vi "Delete TEMP FP Labels.vi"(8 "error in":errorcluster, 11 "owner VI":refnum<vi>) -> (0 "error out":errorcluster, 1 "labels found":i32, 3 "owner VI out":refnum<vi>)   [LabVIEW 2021]
doc: "Delete the temporary front panel labels (not intended to be part of the UI but as a way to distinguish what is going on. This will remove them all by identifying by their tag data.\n\n<b>Code Developed By:</b>\nTechnology Service Corporation\nwww.tsc.com/atcs\n\nDeveloper:\nDaniel Coons"
uses:
  <vilib>/Utility/traverseref.llb/TRef TravTarget.ctl
  <vilib>/Utility/traverseref.llb/VI Scripting - Traverse.lvlib
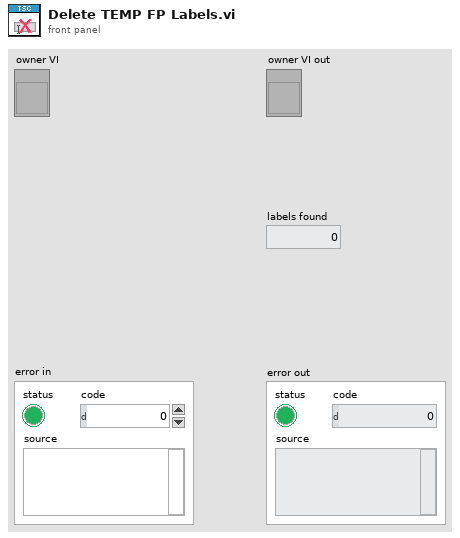
[diagram p1: front panel]
types:
  T1 = typedef "TRef TravTarget.ctl" = enum16{"FP", "BD", "Other"}
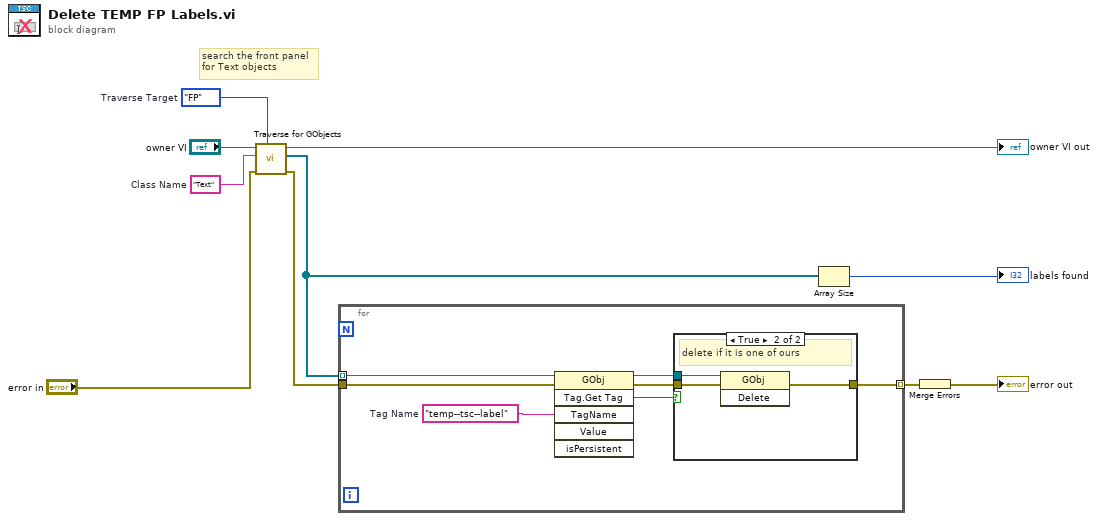
[diagram p0: block diagram]
diagram:
  w9 = TRef_TravTarget."FP"  # Traverse Target
  w10 = "Text"  # Class Name
  # "search the front panel\nfor Text objects"
  n1 = call <vilib>:"Traverse for GObjects.vi"("Traverse Target"=w9, "error in (no error)"="error in", "Class Name"=w10, "VI Refnum"="owner VI") -> ("error out"=w6:errorcluster, "References"=w7:refnum<vi>[], "dup VI Refnum"=→"owner VI out":refnum<vi>)  [unwired: 4 in, 1 out]
  n2 = for {
    tunnel: w7 -> [w16] mode=indexing
    tunnel: w6 -> [w15]
    tunnel: [w13] -> w5 mode=indexing
    w17 = "temp--tsc--label"  # Tag Name
    n3 = invoke class="GObj" method="Tag.Get Tag"(reference=w16, error in=w15, "TagName"=w17) -> (reference out=w12:refnum<vi>, error out=w14:errorcluster, "GetTag"=w11:bool)  [unwired: 3 in, 3 out]
    n4 = case shown="True" w11 {
      tunnel: w14 -> [w18 w21]
      tunnel: [w18 w20] -> w13
      tunnel: w12 -> [_ w19]
      frame False {
      }
      frame True {
        # "delete if it is one of ours"
        n5 = invoke class="GObj" method="Delete"(reference=w19, error in=w21) -> (error out=w20:errorcluster)  [unwired: 1 in, 2 out]
      }
    }
  }
  n6 = Array Size(array=w7) -> (size(s)=→"labels found":i32)
  n7 = Merge Errors(w5) -> (→"error out":errorcluster)
